vi "Resume.vi"(8 "error in (no error)":errorcluster, 11 "VISA resource name":refnum<visa-resource-name>) -> (0 "error out":errorcluster, 3 "VISA resource name out":refnum<visa-resource-name>)   [LabVIEW 2020, in "QuPMXdriver.lvlib"]
doc: "Returns the internal timer value in seconds."
uses:
  QuPMXdriver.lvlib
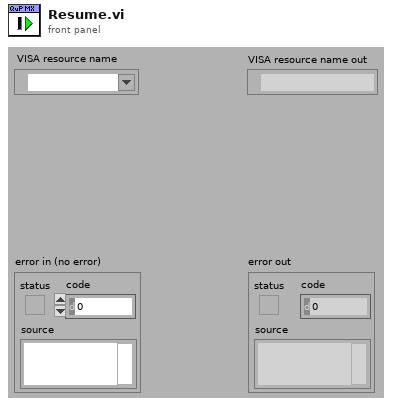
[diagram p1: front panel]
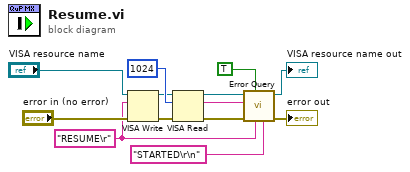
[diagram p0: block diagram]
diagram:
  w4 = "RESUME\r"
  n1 = VISA Write(VISA resource name="VISA resource name", write buffer=w4, error in (no error)="error in (no error)") -> (VISA resource name out=w8:refnum<visa-resource-name>, error out=w1:errorcluster)  [unwired: 1 out]
  n2 = VISA Read(VISA resource name=w8, byte count=u32 1024, error in (no error)=w1) -> (VISA resource name out=w6:refnum<visa-resource-name>, read buffer=w2:string, error out=w5:errorcluster)  [unwired: 1 out]
  n3 = call "Error Query.vi"("Expected read buffer"="STARTED\r\n" ("read buffer"), "Last command"=w4, "Ignore empty sequence? (T)"=TRUE, "error in (no error)"=w5, "Read buffer"=w2, "VISA resource name"=w6) -> ("error out"=→"error out":errorcluster, "VISA resource name out"=→"VISA resource name out":refnum<visa-resource-name>)  [unwired: 4 in]
